vi "Support_TimerStop.vi"(5 "error in (no error)":errorcluster, 7 "Start time":u32) -> (16 "Time (ms)":u32, 19 "error out":errorcluster)   [LabVIEW 2017]
doc: "Calculates time difference."
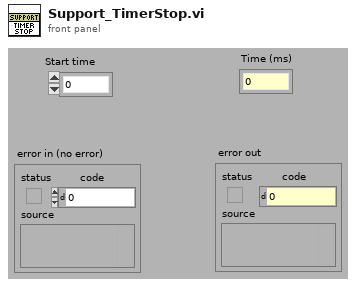
[diagram p1: front panel]
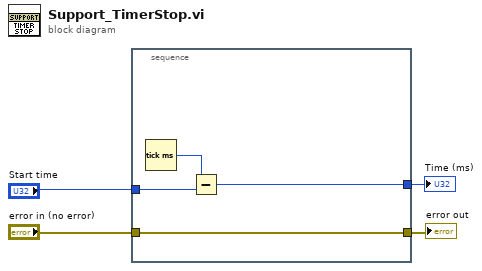
[diagram p0: block diagram]
diagram:
  n1 = stacked-sequence {
    tunnel: [w8] -> w3
    tunnel: "error in (no error)" -> [w8]
    tunnel: "Start time" -> [w6]
    tunnel: [w5] -> w1
    frame #0 {
      n2 = Tick Count (ms)() -> (millisecond timer value=w7:u32)
      n3 = Subtract(x=w7, y=w6) -> (x-y=w5:u32)
    }
  }
  "error out" <- w3
  "Time (ms)" <- w1
